vi "Validate ROI.vi"(9 "ROI in":T1, 10 "SensorHeight_pixels":u32, 11 "SensorWidth_pixels":u32) -> (3 "ROI out":T1)   [LabVIEW 2020]
uses:
  Controls/Region of Interest.ctl
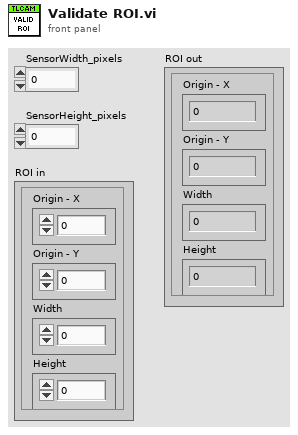
[diagram p1: front panel]
types:
  T1 = typedef "Region of Interest.ctl" = cluster{"Origin - X":u32, "Origin - Y":u32, "Width":u32, "Height":u32}
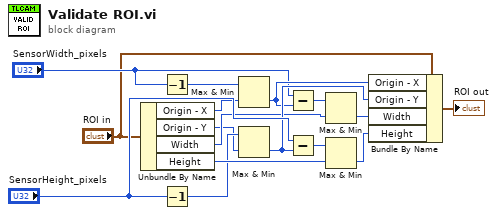
[diagram p0: block diagram]
diagram:
  n1 = Unbundle By Name("ROI in") -> ("Origin - X"=w3:u32, "Origin - Y"=w1:u32, "Width"=w6:u32, "Height"=w10:u32)
  n2 = Decrement(x="SensorWidth_pixels") -> (x-1=w4:u32)
  n3 = Decrement(x="SensorHeight_pixels") -> (x-1=w2:u32)
  n4 = Max & Min(x=w4, y=w3) -> (min(x,y)=w8:u32)  [unwired: 1 out]
  n5 = Max & Min(x=w2, y=w1) -> (min(x,y)=w11:u32)  [unwired: 1 out]
  n6 = Subtract(x="SensorWidth_pixels", y=w8) -> (x-y=w9:u32)
  n7 = Subtract(x="SensorHeight_pixels", y=w11) -> (x-y=w13:u32)
  n8 = Max & Min(x=w9, y=w6) -> (min(x,y)=w14:u32)  [unwired: 1 out]
  n9 = Max & Min(x=w13, y=w10) -> (min(x,y)=w15:u32)  [unwired: 1 out]
  n10 = Bundle By Name(cluster="ROI in", "Origin - X"=w8, "Origin - Y"=w11, "Width"=w14, "Height"=w15) -> (→"ROI out":T1)
